vi "Teleop.vi"(10 "Match Info":T1={"Autonomous Elapsed Seconds"=0.0, "TeleOp Elapsed Seconds"=0.0, "Disabled Elapsed Seconds"=0.0, "Visited Autonomous"=FALSE, "Visited TeleOp"=FALSE, "Visited Disabled"=FALSE, "Autonomous Settings"={"Autonomous Style"=enum."Independent", "VI Refnum"=refnum}}, 11 "Call Context":T2) -> ()   [LabVIEW 2013]
doc: "This VI is called for each TeleOp packet received from the DS where the robot is not disabled. It is often used to read from the joysticks and update I/O or to update setpoints for timed control loops. It should complete and return within 20 milliseconds or it may miss DS packets."
uses:
  <vilib>/Rock Robotics/WPI/DriverStation/WPI_DriverStationDerivedRobotMode.ctl
  <vilib>/Rock Robotics/WPI/DriverStation/WPI_DriverStationMatch Info.ctl
  <vilib>/Rock Robotics/WPI/Solenoid/WPI_SolenoidValue.ctl
  Robot Global Data.vi
  <vilib>/Rock Robotics/WPI/Solenoid/Deprecated/WPI_SolenoidGetBool.vi
  <vilib>/Rock Robotics/WPI/Solenoid/WPI_SolenoidSetEnum.vi
  <vilib>/Rock Robotics/WPI/Joystick/WPI_JoystickGetSetRefNum.vi
  <vilib>/Rock Robotics/WPI/RobotDrive/WPI_RobotDriveGetSetRefNum.vi
panel:
  out "Voltage":dbl
  out "Value":bool
  out "Ultrasoic Value":dbl
  out "Numeric 1":dbl(slide) scale=0.0..100.0
  out "Boolean 2":bool
  out "Boolean 1":bool
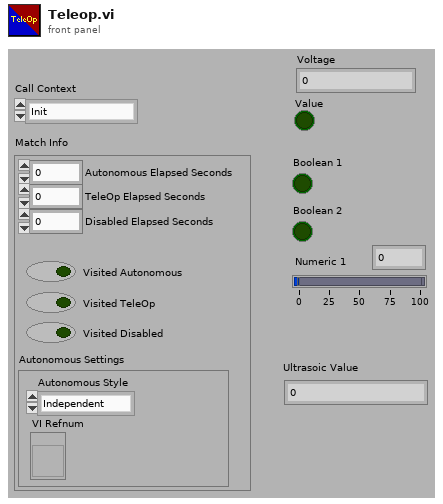
[diagram p1: front panel]
types:
  T1 = typedef "WPI_DriverStationMatch Info.ctl" = cluster{"Autonomous Elapsed Seconds":dbl, "TeleOp Elapsed Seconds":dbl, "Disabled Elapsed Seconds":dbl, "Visited Autonomous":bool, "Visited TeleOp":bool, "Visited Disabled":bool, "Autonomous Settings":cluster{"Autonomous Style":enum16{"Iterative", "Independent"}, "VI Refnum":refnum<vi>}}
  T2 = typedef "WPI_DriverStationDerivedRobotMode.ctl" = enum16{"Init", "Execute", "Stop"}
  T3 = typedef "WPI_RobotDriveDevRef.ctl" = cluster{"DevStatus":errorcluster, "Motors[]":T4[], "Square Inputs":bool, "Max Output":dbl, "Isochronous":bool}
  T4 = typedef "WPI_MotorControlDeviceRef.ctl" = cluster{"DeviceStatus":errorcluster, "Type":enum16{"PWM", "CAN"}, "PWM":cluster{"Digital Module":T5, "PWM Channel":T6, "DeadBand":T7}, "CAN":cluster{"Device Number":u8, "Control Mode":T8, "Semaphore":T9, "Max Vout":dbl}, "Invert":bool, "TransformRef":T10, "InvTransformRef":T10}
  T5 = typedef "FPGA_TypedefDigitalModule.ctl" = enum16{"Digital Module 1", "Digital Module 2"}
  T6 = typedef "FPGA_DIOPWMChannel.ctl" = enum8{"PWM 1", "PWM 2", "PWM 3", "PWM 4", "PWM 5", "PWM 6", "PWM 7", "PWM 8", "PWM 9", "PWM 10", "Invalid"}
  T7 = typedef "WPI_PWMDeadband.ctl" = cluster{"Name":string, "maxPositivePwm":i32, "minPositivePwm":i32, "centerPwm":i32, "maxNegativePwm":i32, "minNegativePwm":i32, "angularRange":u16}
  T8 = typedef "WPI_CANJaguar_ControlMode.ctl" = enum8{"Percent VBus", "Current", "Speed", "Position", "Voltage"}
  T9 = typedef "Semaphore RefNum" = refnum<k1>
  T10 = typedef "WPI_PWMTransform_ConPane.ctl" = refnum<vi>
  T11 = typedef "WPI_JoystickDevRef.ctl" = cluster{"Device":T12}
  T12 = typedef "WPI_JoystickDeviceEnum.ctl" = enum16{"USB 1", "USB 2", "USB 3", "USB 4", "Kinect 1", "Kinect 2"}
  T13 = typedef "WPI_AnalogChannelDevRef.ctl" = cluster{"DevStatus":errorcluster, "Analog Module":T14, "Analog Channel":T15}
  T14 = typedef "FPGA_TypedefAnalogModule.ctl" = enum16{"Analog Module 1", "Analog Module 2"}
  T15 = typedef "FPGA_AIChannel.ctl" = enum8{"AI 1", "AI 2", "AI 3", "AI 4", "AI 5", "AI 6", "AI 7", "AI 8", "Invalid"}
  T16 = typedef "WPI_RelayDevRef.ctl" = cluster{"DevStatus":errorcluster, "Relay Channel":T17, "Digital Module":T5, "Relay Direction":T18}
  T17 = typedef "FPGA_DIORelayChannel.ctl" = enum8{"Relay 1", "Relay 2", "Relay 3", "Relay 4", "Relay 5", "Relay 6", "Relay 7", "Relay 8", "Invalid"}
  T18 = typedef "WPI_RelayDirection.ctl" = enum16{"Both directions", "Forward only", "Reverse only"}
  T19 = typedef "WPI_JoystickButtonState.ctl" = cluster{"Button 1":bool, "Button 2":bool, "Button 3":bool, "Button 4":bool, "Button 5":bool, "Button 6":bool, "Button 7":bool, "Button 8":bool, "Button 9":bool, "Button 10":bool, "Button 11":bool, "Button 12":bool}
  T20 = cluster{"axis 1 (x)":dbl, "axis 2 (y)":dbl, "axis 3 (throttle)":dbl, "axis 4":dbl, "axis 5":dbl, "axis 6":dbl}
  T21 = typedef "WPI_DigitalInputDevRef.ctl" = cluster{"DevStatus":errorcluster, "DIO Channel":T22, "Digital Module":T5}
  T22 = typedef "FPGA_DIOChannel.ctl" = enum8{"DIO 1", "DIO 2", "DIO 3", "DIO 4", "DIO 5", "DIO 6", "DIO 7", "DIO 8", "DIO 9", "DIO 10", "DIO 11", "DIO 12", "DIO 13", "DIO 14", "Invalid"}
  T23 = typedef "WPI_SolenoidDevRef.ctl" = cluster{"DevStatus":errorcluster, "Solenoid Module":T24, "Forward Solenoid Channel":T25, "Reverse Solenoid Channel":T25}
  T24 = typedef "FPGA_TypedefSolenoidModule.ctl" = enum16{"Solenoid Module 1", "Solenoid Module 2"}
  T25 = typedef "WPI_SolenoidChannel.ctl" = enum8{"Solenoid 1", "Solenoid 2", "Solenoid 3", "Solenoid 4", "Solenoid 5", "Solenoid 6", "Solenoid 7", "Solenoid 8", "Invalid"}
  T26 = typedef "WPI_SolenoidValue.ctl" = enum16{"Off", "On", "Forward", "Reverse"}
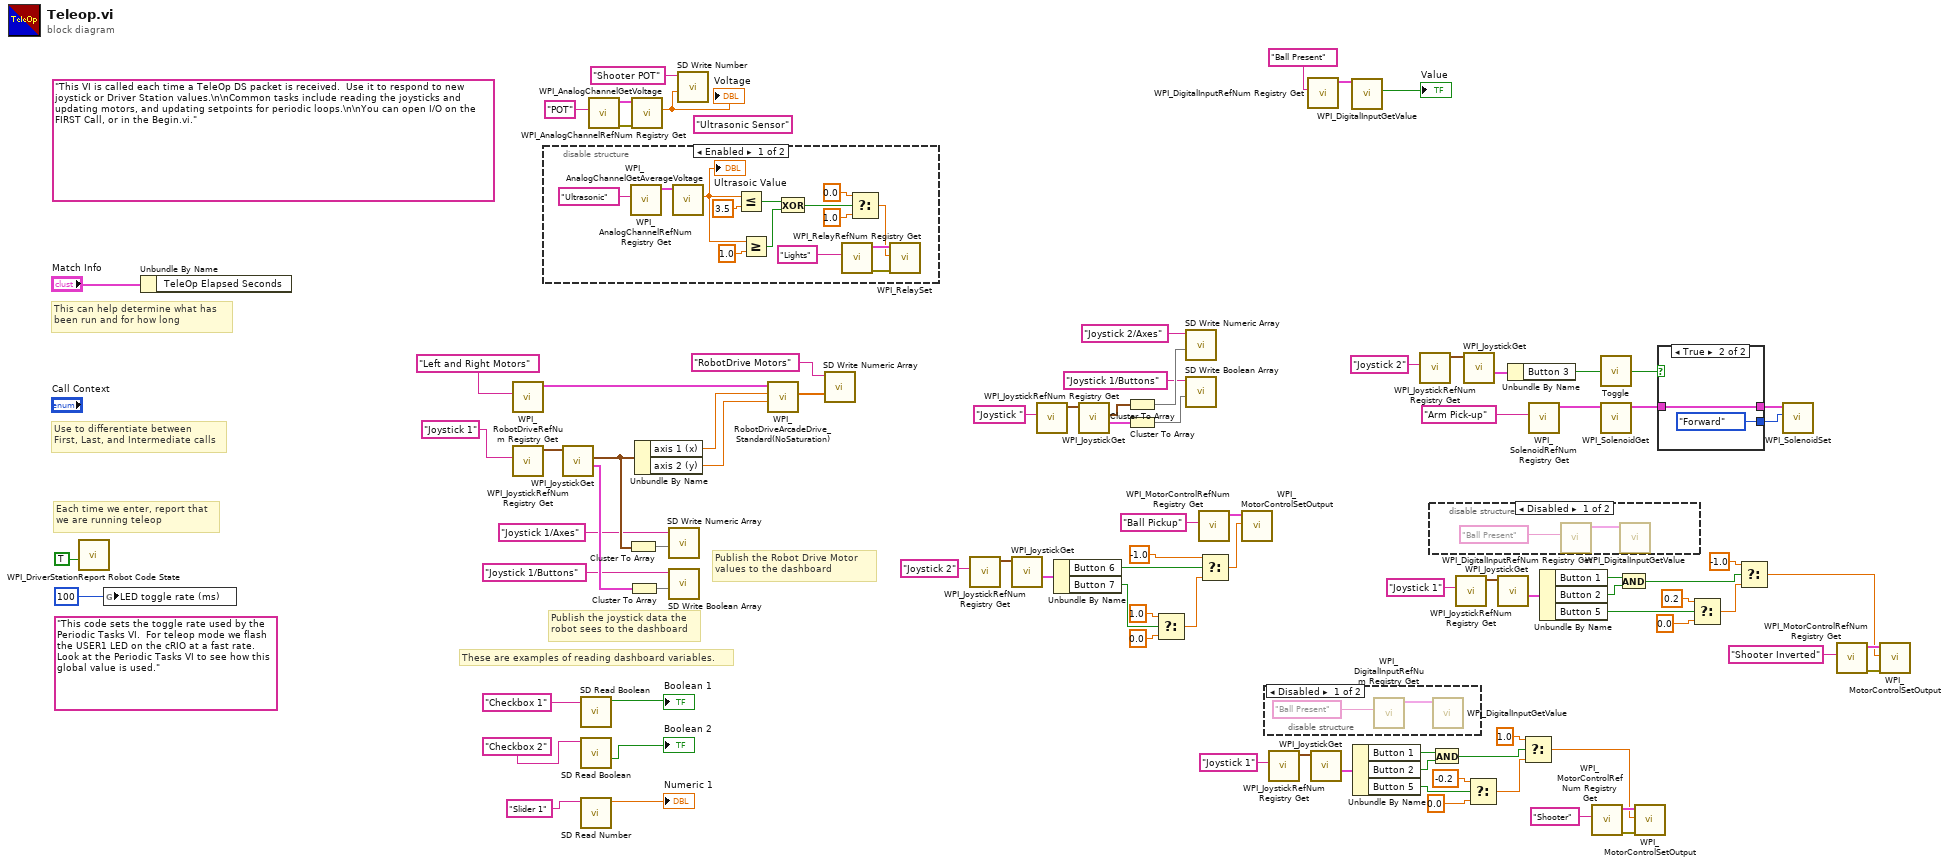
[diagram p0: block diagram]
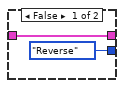
[diagram p5: hidden frame]
diagram:
  (unwired) "Ultrasonic Sensor" ("Name")
  (unwired) "This code sets the toggle rate used by the Periodic Tasks VI.  For teleop mode we flash the USER1 LED on the cRIO at a fast rate.  Look at the Periodic Tasks VI to see how this global value is used."
  (unwired) "This VI is called each time a TeleOp DS packet is received.  Use it to respond to new joystick or Driver Station values.\n\nCommon tasks include reading the joysticks and updating motors, and updating setpoints for periodic loops.\n\nYou can open I/O on the FIRST Call, or in the Begin.vi."
  # "These are examples of reading dashboard variables."
  # "Publish the Robot Drive Motor\nvalues to the dashboard"
  # "Publish the joystick data the\nrobot sees to the dashboard"
  # "Each time we enter, report that\nwe are running teleop"
  # "Use to differentiate between\nFirst, Last, and Intermediate calls"
  # "This can help determine what has\nbeen run and for how long"
  n1 = call <vilib>:"WPI_DriverStationReport Robot Code State.vi"("TeleOp"=TRUE ("Autonomous")) -> ()  [unwired: 10 in, 1 out]
  n2 = global write "Robot Global Data.vi" "LED toggle rate (ms)"(u32 100 ("LED ms toggle rate")) -> ()
  n3 = Unbundle By Name("Match Info") -> ()  [unwired: 1 out]
  n4 = call <vilib>:"WPI_RobotDriveRefNum Registry Get.vi"("refnum name"="Left and Right Motors") -> ("RobotDriveDevRef"=w89:T3)  [unwired: 1 in, 9 out]
  n5 = call <vilib>:"WPI_JoystickRefNum Registry Get.vi"("refnum name"="Joystick 1") -> ("JoystickDevRef"=w85:T11)  [unwired: 1 in, 9 out]
  n6 = disable-structure shown="Enabled" {
    frame Enabled {
      n7 = call <vilib>:"WPI_AnalogChannelRefNum Registry Get.vi"("refnum name"="Ultrasonic") -> ("AIDeviceRef"=w104:T13)  [unwired: 9 in, 1 out]
      n8 = call <vilib>:"WPI_AnalogChannelGetAverageVoltage.vi"("AIDeviceRef"=w104) -> ("Voltage"=w103:dbl)  [unwired: 8 in, 2 out]
      "Ultrasoic Value" <- w103
      n9 = Less Or Equal?(x=w103, y=3.5) -> (x <= y?=w100:bool)
      n10 = Greater Or Equal?(x=w103, y=1.0) -> (x >= y?=w99:bool)
      n11 = Exclusive Or(1:w99, 2:w100) -> (0:w98:bool)
      n12 = call <vilib>:"WPI_RelayRefNum Registry Get.vi"("refnum name"="Lights") -> ("error out"=w95:errorcluster, "RelayDevRef"=w94:T16)  [unwired: 9 in]
      n13 = Select(t=0.0, s=w98, f=1.0) -> (s? t:f=w93:dbl)
      n14 = call <vilib>:"WPI_RelaySet.vi"("error in (no error)"=w95, "RelayValue"=w93, "RelayDevRef"=w94) -> ()  [unwired: 7 in, 2 out]
    }
    frame Disabled {
    }
  }
  n15 = call <vilib>:"WPI_JoystickGet.vi"("JoystickDevRef"=w85) -> ("Buttons"=w82:T19, "Axes"=w79:T20)  [unwired: 1 in, 4 out]
  n16 = call <vilib>:"SD Read Boolean.vi"("Name"="Checkbox 1" ("refnum name")) -> ("Boolean"=→"Boolean 1":bool)  [unwired: 8 in, 2 out]
  n17 = call <vilib>:"SD Read Boolean.vi"("Name"="Checkbox 2" ("refnum name")) -> ("Boolean"=→"Boolean 2":bool)  [unwired: 8 in, 2 out]
  n18 = call <vilib>:"SD Read Number.vi"("Name"="Slider 1" ("refnum name")) -> ("Numeric"=→"Numeric 1":dbl)  [unwired: 8 in, 2 out]
  n19 = call <vilib>:"WPI_AnalogChannelRefNum Registry Get.vi"("refnum name"="POT") -> ("error out"=w25:errorcluster, "AIDeviceRef"=w26:T13)  [unwired: 9 in]
  n20 = Cluster To Array(cluster=w79) -> (array=w78:dbl[])
  n21 = Cluster To Array(cluster=w82) -> (array=w81:bool[])
  n22 = call <vilib>:"WPI_AnalogChannelGetVoltage.vi"("error in (no error)"=w25, "AIDeviceRef"=w26) -> ("Voltage"=w23:dbl)  [unwired: 7 in, 2 out]
  "Voltage" <- w23
  n23 = Unbundle By Name(w79) -> ("axis 1 (x)"=w88:dbl, "axis 2 (y)"=w87:dbl)
  n24 = call <vilib>:"SD Write Numeric Array.vi"("Numeric Array"=w78, "Name"="Joystick 1/Axes") -> ()  [unwired: 8 in, 2 out]
  n25 = call <vilib>:"SD Write Boolean Array.vi"("Boolean Array"=w81, "Name"="Joystick 1/Buttons") -> ()  [unwired: 8 in, 2 out]
  n26 = call <vilib>:"SD Write Number.vi"("Numeric"=w23, "Name"="Shooter POT" ("Table Prefix out")) -> ()  [unwired: 8 in, 2 out]
  n27 = call <vilib>:"WPI_RobotDriveArcadeDrive_Standard(NoSaturation).vi"("Y axis value"=w87, "X axis value"=w88, "RobotDriveDevRef"=w89) -> ("Motor Values"=w75:dbl[])  [unwired: 1 in, 7 out]
  n28 = call <vilib>:"SD Write Numeric Array.vi"("Numeric Array"=w75, "Name"="RobotDrive Motors") -> ()  [unwired: 8 in, 2 out]
  n29 = call <vilib>:"WPI_JoystickRefNum Registry Get.vi"("refnum name"="Joystick 2") -> ("JoystickDevRef"=w52:T11)  [unwired: 9 in, 1 out]
  n30 = call <vilib>:"WPI_JoystickGet.vi"("JoystickDevRef"=w52) -> ("Buttons"=w53:T19)  [unwired: 4 in, 2 out]
  n31 = call <vilib>:"WPI_JoystickRefNum Registry Get.vi"("refnum name"="Joystick ") -> ("JoystickDevRef"=w15:T11)  [unwired: 1 in, 9 out]
  n32 = Unbundle By Name(w53) -> ("Button 6"=w54:bool, "Button 7"=w50:bool)
  n33 = call <vilib>:"WPI_JoystickGet.vi"("JoystickDevRef"=w15) -> ("Buttons"=w16:T19, "Axes"=w19:T20)  [unwired: 1 in, 4 out]
  n34 = Cluster To Array(cluster=w19) -> (array=w20:dbl[])
  n35 = Cluster To Array(cluster=w16) -> (array=w17:bool[])
  n36 = Select(t=1.0, s=w50, f=0.0) -> (s? t:f=w2:dbl)
  n37 = call <vilib>:"SD Write Numeric Array.vi"("Numeric Array"=w20, "Name"="Joystick 2/Axes") -> ()  [unwired: 8 in, 2 out]
  n38 = call <vilib>:"SD Write Boolean Array.vi"("Boolean Array"=w17, "Name"="Joystick 1/Buttons") -> ()  [unwired: 8 in, 2 out]
  n39 = call <vilib>:"WPI_MotorControlRefNum Registry Get.vi"("refnum name"="Ball Pickup") -> ("MotorControlDevRef"=w58:T4)  [unwired: 9 in, 1 out]
  n40 = Select(t=-1.0, s=w54, f=w2) -> (s? t:f=w1:dbl)
  n41 = call <vilib>:"WPI_MotorControlSetOutput.vi"("Output"=w1, "MotorControlDevRef"=w58) -> ()  [unwired: 7 in, 3 out]
  n42 = disable-structure shown="Disabled" {
    frame Disabled {
      n43 = call <vilib>:"WPI_DigitalInputRefNum Registry Get.vi"("refnum name"="Ball Present") -> ("DigitalInputDevRef"=w107:T21)  [unwired: 9 in, 1 out]
      n44 = call <vilib>:"WPI_DigitalInputGetValue.vi"("DigitalInputDevRef"=w107) -> ()  [unwired: 8 in, 3 out]
    }
    frame Enabled {
    }
  }
  n45 = call <vilib>:"WPI_JoystickRefNum Registry Get.vi"("refnum name"="Joystick 1") -> ("JoystickDevRef"=w67:T11)  [unwired: 9 in, 1 out]
  n46 = call <vilib>:"WPI_DigitalInputRefNum Registry Get.vi"("refnum name"="Ball Present") -> ("DigitalInputDevRef"=w12:T21)  [unwired: 9 in, 1 out]
  n47 = call <vilib>:"WPI_JoystickGet.vi"("JoystickDevRef"=w67) -> ("Buttons"=w66:T19)  [unwired: 4 in, 2 out]
  n48 = call <vilib>:"WPI_DigitalInputGetValue.vi"("DigitalInputDevRef"=w12) -> ("Value"=→"Value":bool)  [unwired: 8 in, 2 out]
  n49 = Unbundle By Name(w66) -> ("Button 1"=w33:bool, "Button 2"=w32:bool, "Button 5"=w30:bool)
  n50 = call <vilib>:"WPI_JoystickRefNum Registry Get.vi"("refnum name"="Joystick 2") -> ("JoystickDevRef"=w47:T11)  [unwired: 9 in, 1 out]
  n51 = disable-structure shown="Disabled" {
    frame Disabled {
      n52 = call <vilib>:"WPI_DigitalInputRefNum Registry Get.vi"("refnum name"="Ball Present") -> ("DigitalInputDevRef"=w108:T21)  [unwired: 9 in, 1 out]
      n53 = call <vilib>:"WPI_DigitalInputGetValue.vi"("DigitalInputDevRef"=w108) -> ()  [unwired: 8 in, 3 out]
    }
    frame Enabled {
    }
  }
  n54 = And(x=w33, y=w32) -> (x .and. y?=w5:bool)
  n55 = call <vilib>:"WPI_JoystickRefNum Registry Get.vi"("refnum name"="Joystick 1") -> ("JoystickDevRef"=w61:T11)  [unwired: 9 in, 1 out]
  n56 = call <vilib>:"WPI_JoystickGet.vi"("JoystickDevRef"=w47) -> ("Buttons"=w46:T19)  [unwired: 4 in, 2 out]
  n57 = Select(t=-0.2, s=w30, f=0.0) -> (s? t:f=w4:dbl)
  n58 = call <vilib>:"WPI_JoystickGet.vi"("JoystickDevRef"=w61) -> ("Buttons"=w62:T19)  [unwired: 4 in, 2 out]
  n59 = Unbundle By Name(w46) -> ("Button 3"=w40:bool)
  n60 = Select(t=1.0, s=w5, f=w4) -> (s? t:f=w3:dbl)
  n61 = call <vilib>:"WPI_SolenoidRefNum Registry Get.vi"("refnum name"="Arm Pick-up") -> ("SolenoidDevRef"=w45:T23)  [unwired: 9 in, 1 out]
  n62 = Unbundle By Name(w62) -> ("Button 1"=w34:bool, "Button 2"=w35:bool, "Button 5"=w31:bool)
  n63 = call <vilib>:"WPI_MotorControlRefNum Registry Get.vi"("refnum name"="Shooter") -> ("error out"=w64:errorcluster, "MotorControlDevRef"=w63:T4)  [unwired: 9 in]
  n64 = call "Toggle.vi"("Input"=w40) -> ("Toggled Output"=w44:bool)
  n65 = call-poly <vilib>:"WPI_SolenoidGet.vi"("SolenoidDevRef"=w45) -> ("SolenoidDevRef"=w43:T23)  [unwired: 8 in, 2 out]
  n66 = And(x=w34, y=w35) -> (x .and. y?=w9:bool)
  n67 = call <vilib>:"WPI_MotorControlSetOutput.vi"("error in (no error)"=w64, "Output"=w3, "MotorControlDevRef"=w63) -> ()  [unwired: 6 in, 3 out]
  n68 = case shown="True" w44 {
    tunnel: w43 -> [w111 w113]
    tunnel: [w111 w113] -> w42
    tunnel: [WPI_SolenoidValue."Reverse" ("Value") WPI_SolenoidValue."Forward" ("Value")] -> w41
    frame False {
    }
    frame True {
    }
  }
  n69 = Select(t=0.2, s=w31, f=0.0) -> (s? t:f=w8:dbl)
  n70 = Select(t=-1.0, s=w9, f=w8) -> (s? t:f=w7:dbl)
  n71 = call-poly <vilib>:"WPI_SolenoidSet.vi"("Value"=w41, "SolenoidDevRef"=w42) -> ()  [unwired: 8 in, 2 out]
  n72 = call <vilib>:"WPI_MotorControlRefNum Registry Get.vi"("refnum name"="Shooter Inverted") -> ("error out"=w28:errorcluster, "MotorControlDevRef"=w29:T4)  [unwired: 9 in]
  n73 = call <vilib>:"WPI_MotorControlSetOutput.vi"("error in (no error)"=w28, "Output"=w7, "MotorControlDevRef"=w29) -> ()  [unwired: 6 in, 3 out]
